vi "Set Sector.vi"(9 "Numeric":i32, 11 "PN532 COM Port":refnum<visa-resource-name>) -> (0 "Error Out":errorcluster, 3 "PN532 COM out":refnum<visa-resource-name>)   [LabVIEW 2012, in "NFC Driver.lvlib"]
doc: "This VI writes to the NTAG's memory the data contained in \"Data to write (max 16 bytes)\" to the page specified in \"Page\".\n\nThe maximum size of the data to write is 16 bytes or 4 characters. Any data larger than 16 bytes will be truncated."
uses:
  NFC Driver.lvlib
panel:
  out "Selected substring (HEX)":string
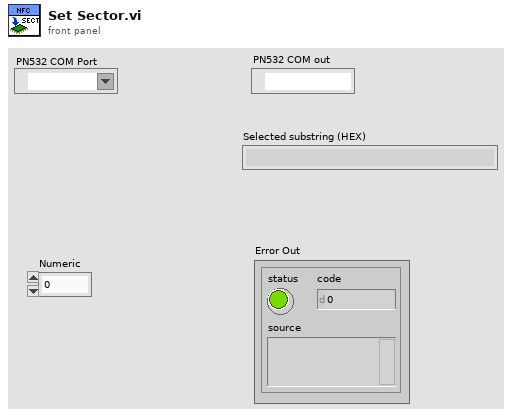
[diagram p1: front panel]
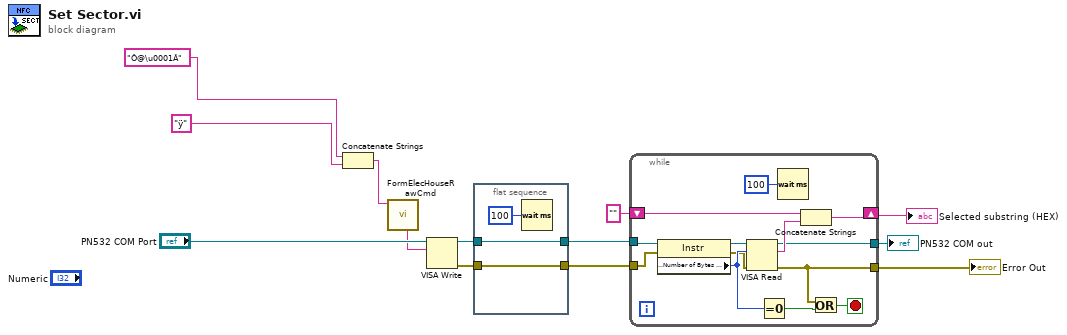
[diagram p0: block diagram]
diagram:
  n1 = Concatenate Strings("Ô@\u0001Â" ("string"), "ÿ" ("string")) -> (w11:string)
  n2 = call "FormElecHouseRawCmd.vi"("Command"=w11) -> ("concatenated Cmd"=w12:string)  [unwired: 10 in]
  n3 = VISA Write(VISA resource name="PN532 COM Port", write buffer=w12) -> (VISA resource name out=w10:refnum<visa-resource-name>, error out=w9:errorcluster)  [unwired: 1 in, 1 out]
  n4 = flat-sequence {
    tunnel: w10 -> [w15]
    tunnel: [w15] -> w5
    tunnel: w9 -> [w14]
    tunnel: [w14] -> w7
    frame #0 {
      n5 = Wait (ms)(milliseconds to wait=u32 100) -> ()  [unwired: 1 out]
    }
  }
  n6 = while {
    tunnel: w5 -> [w29]
    tunnel: w7 -> [w22]
    shift-right: [w23] -> w3
    shift-left: "" -> [w25]
    tunnel: [w18] -> w6
    tunnel: [w17] -> w1
    stop <- w19 stop-if-true
    n7 = property class="Instr"(reference=w29, error in=w22) -> (reference out=w28:refnum<visa-resource-name>, error out=w21:errorcluster, "Serial Settings:Number of Bytes at Serial Port"=w27:u32)
    n8 = VISA Read(VISA resource name=w28, byte count=w27, error in (no error)=w21) -> (VISA resource name out=w17:refnum<visa-resource-name>, read buffer=w24:string, error out=w18:errorcluster)  [unwired: 1 out]
    n9 = Equal To 0?(x=w27) -> (x = 0?=w20:bool)
    n10 = Wait (ms)(milliseconds to wait=u32 100) -> ()  [unwired: 1 out]
    n11 = Concatenate Strings(w25, w24) -> (w23:string)
    n12 = Or(x=w18, y=w20) -> (x .or. y?=w19:bool)
  }
  "Error Out" <- w6
  "Selected substring (HEX)" <- w3
  "PN532 COM out" <- w1
